vi "Write Name Dependecy.vi"(8 "error in (no error)":errorcluster, 10 "Name Dependecy":i32, 11 "Mapping Column in":refnum<class "Mapping Column.lvclass">) -> (0 "error out":errorcluster, 3 "Mapping Column out":refnum<class "Mapping Column.lvclass">)   [LabVIEW 2013, in "Table Manager.lvlib" / "Mapping Column.lvclass"]
uses:
  Mapping Column.lvclass
  Mapping Column.lvclass/Mapping Column.ctl
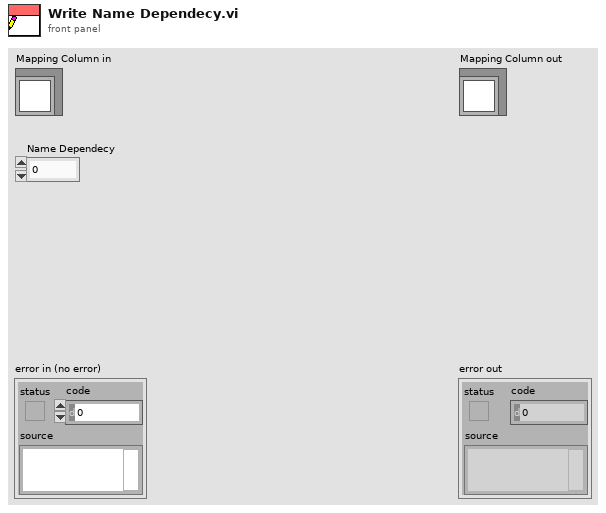
[diagram p1: front panel]
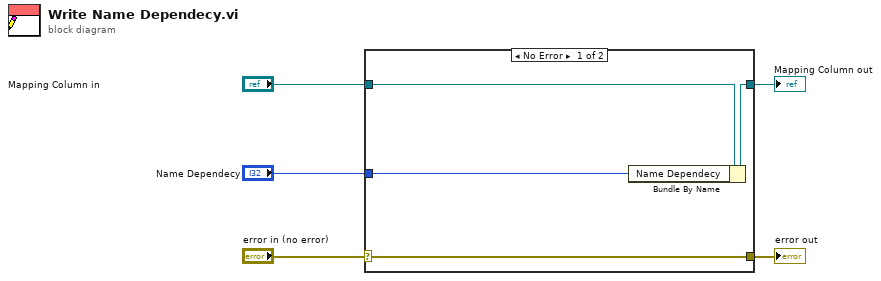
[diagram p0: block diagram]
diagram:
  n1 = case shown="No Error" "error in (no error)" {
    selector: "error in (no error)" -> [w9 w10]
    tunnel: [w9 w10] -> w4
    tunnel: [w7 w11] -> w2
    tunnel: "Mapping Column in" -> [w8 w11]
    tunnel: "Name Dependecy" -> [w6 _]
    frame No Error {
      n2 = Bundle By Name(cluster=w8, "Name Dependecy"=w6) -> (w7:refnum<class "Mapping Column.lvclass">)
    }
    frame Error {
    }
  }
  "error out" <- w4
  "Mapping Column out" <- w2
